vi "Waveform Channel Level.vi"(8 "error in (no error)":errorcluster, 11 "Node Ptr":T1 format="%.0x") -> (0 "error out":errorcluster)   [LabVIEW 2023, in "Embedded TDMS Logger System Explorer.lvlib"]
uses:
  Embedded TDMS Logger System Explorer.lvlib
  <vilib>/NI VeriStand/Custom Device API/Custom Device Item Ref.ctl
  Shared/Meta Data Item.ctl
  <vilib>/NI VeriStand/Custom Device API/Get Item Property (Dependent Node Pointer).vi
  <vilib>/NI VeriStand/Custom Device API/Set Item Property (Dependent Node Pointer).vi
  <vilib>/NI VeriStand/Custom Device API/Get Item Property (Variant).vi
  <vilib>/NI VeriStand/Custom Device API/Set Item Property (Variant).vi
  NationalInstruments.VeriStand.SystemStorage
  <vilib>/NI VeriStand/Custom Device API/Custom Device API.lvlib
  Shared/Embedded TDMS Logger Shared.lvlib
  <vilib>/NI VeriStand/Custom Device Tools/Custom Device Utility Library/Custom Device Utility Library.lvlib
panel:
  in  "Channel":string(combo)
  in  "Group Level Meta Data":string[][](table)
  in  "Specific Header":cluster{"Section Name":string}={"Section Name"="Specific Page Settings"}
  in  "General Header":cluster{"Section Name":string}={"Section Name"="General Page Settings"}
  in  "Description":string
  in  "Channel Name":string
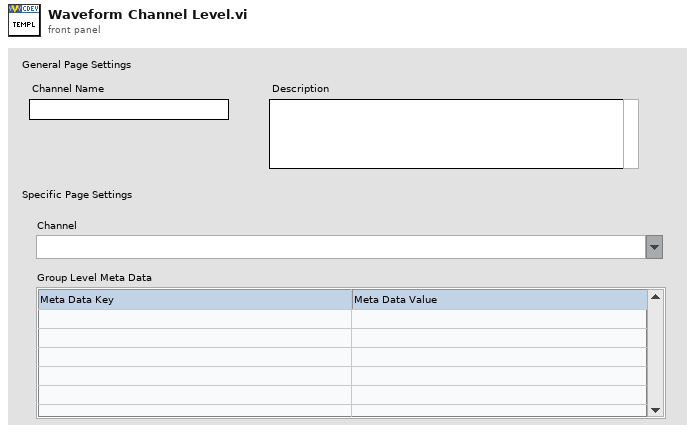
[diagram p1: front panel]
types:
  T1 = typedef "Custom Device API.lvlib/Custom Device Item Ref.ctl" = u64
  T2 = typedef "Embedded TDMS Logger Shared.lvlib/Meta Data Item.ctl" = cluster{"Key":string, "Value":string}
  T3 = typedef "Custom Device API.lvlib/Custom Device Pointer.ctl" = refnum<k24>
  T4 = typedef "Custom Device API.lvlib/Custom Device Item Info.ctl" = cluster{"Name":string, "Is Channel":bool, "GUID":string, "Is Waveform":bool}
  T5 = typedef "Custom Device API.lvlib/Custom Device Commands.ctl" = enum16{"Default", "Item renamed", "Shutdown", "Dynamic button pressed"}
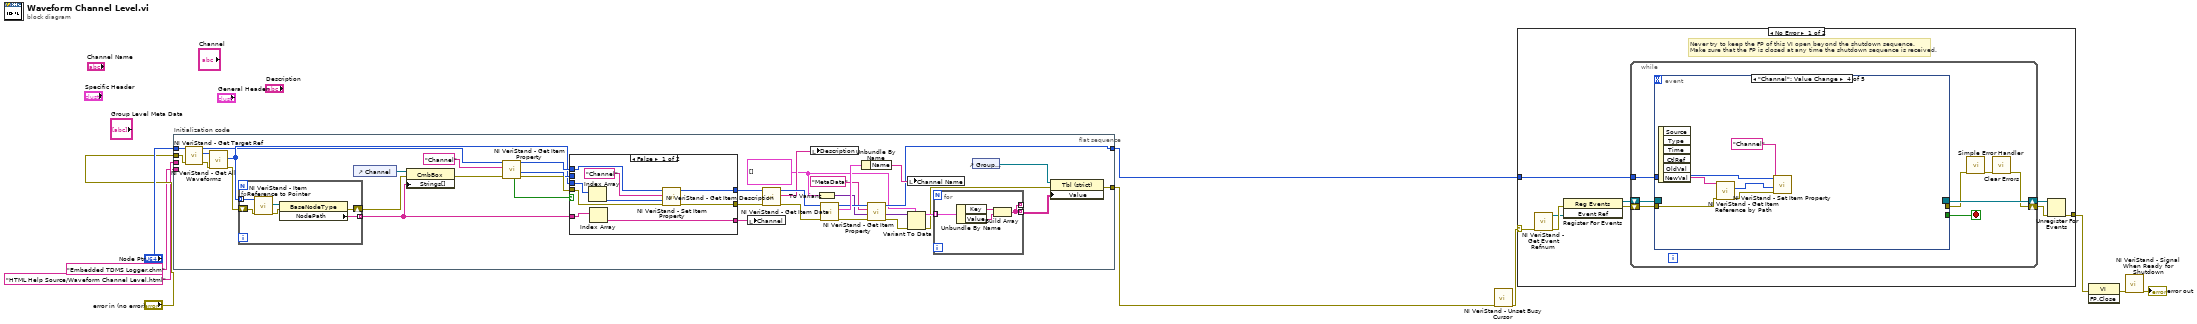
[diagram p0: block diagram]
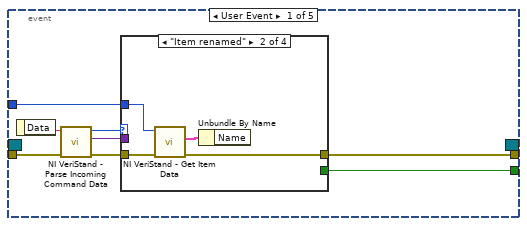
[diagram p2: hidden frame]
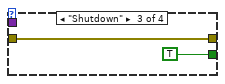
[diagram p4: hidden frame]
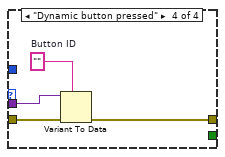
[diagram p5: hidden frame]
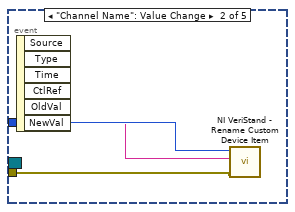
[diagram p6: hidden frame]
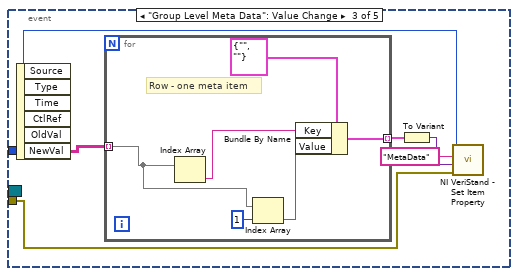
[diagram p7: hidden frame]
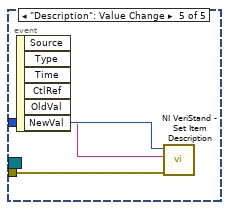
[diagram p8: hidden frame]
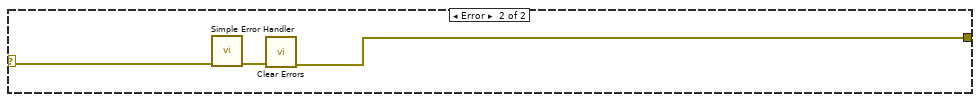
[diagram p9: hidden frame]
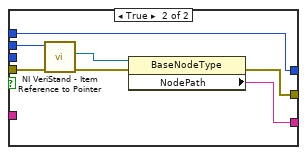
[diagram p10: hidden frame]
diagram:
  n1 = flat-sequence "Initialization code" {
    tunnel: "error in (no error)" -> [w39]
    tunnel: "Node Ptr" -> [w38]
    tunnel: [w24] -> w6
    tunnel: [w33] -> w3
    tunnel: "HTML Help Source/Waveform Channel Level.html" ("CD_CHM_Section") -> [_]
    tunnel: "Embedded TDMS Logger.chm" ("CD_CHM_FileName") -> [_]
    frame #0 {
      w29 = T2[] []
      n2 = call <vilib>:"NI VeriStand - Get Target Ref.vi"("error in"=w39, "Item Ref in"=w38) -> ("error out"=w40:errorcluster, "Target Ref"=w11:T1, "Item Ref out"=w12:T1)  [unwired: 6 in, 1 out]
      n3 = call <vilib>:"NI VeriStand - Get All Waveforms.vi"("error in"=w40, "Section Ref in"=w11) -> ("error out"=w41:errorcluster, "Waveform Refs"=w13:T1[])  [unwired: 6 in, 2 out]
      n4 = for {
        tunnel: w13 -> [w73] mode=indexing
        shift-right: [w68] -> w37
        shift-left: w41 -> [w72]
        tunnel: [w69] -> w18 mode=indexing
        n5 = call <vilib>:"NI VeriStand - Item Reference to Pointer.vi"("error in (no error)"=w72, "Item Ref in"=w73) -> ("error out"=w71:errorcluster, "Node Pointer"=w70:T3)  [unwired: 6 in, 2 out]
        n6 = property class="BaseNodeType"(reference=w70, error in=w71) -> (error out=w68:errorcluster, "NodePath"=w69:string)  [unwired: 1 out]
      }
      n7 = control-ref of="Channel"() -> (w42:refnum<vi>)
      n8 = property class="CmbBox"(reference=w42, error in=w37, "Strings[]"=w18) -> (error out=w14:errorcluster)  [unwired: 1 out]
      n9 = call-poly <vilib>:"NI VeriStand - Get Item Property.vi"("error in (no error)"=w14, "Property Name"="Channel", "Item Ref in"=w12) -> ("error out"=w22:errorcluster, "Dependent Node Ref"=w21:T1, "Item Ref out"=w20:T1, "Found"=w19:bool)  [unwired: 5 in]
      n10 = case shown="False" w19 {
        tunnel: w21 -> [_ w61]
        tunnel: w22 -> [w54 w60]
        tunnel: [w53 w59] -> w16
        tunnel: [w51 w58] -> w17
        tunnel: w20 -> [w55 w57]
        tunnel: w18 -> [w52 _]
        tunnel: [w50 w57] -> w15
        tunnel: w13 -> [w49 _]
        frame False {
          n11 = Index Array(array=w49) -> (element=w48:T1)  [unwired: 1 in]
          n12 = Index Array(array=w52) -> (element=w51:string)  [unwired: 1 in]
          n13 = call-poly <vilib>:"NI VeriStand - Set Item Property.vi"("error in (no error)"=w54, "Dependent Node Ref"=w48, "Property Name"="Channel", "Item Ref in"=w55) -> ("error out"=w53:errorcluster, "Item Ref out"=w50:T1)  [unwired: 5 in, 1 out]
        }
        frame True {
          n14 = call <vilib>:"NI VeriStand - Item Reference to Pointer.vi"("error in (no error)"=w60, "Item Ref in"=w61) -> ("error out"=w62:errorcluster, "Node Pointer"=w63:T3)  [unwired: 6 in, 2 out]
          n15 = property class="BaseNodeType"(reference=w63, error in=w62) -> (error out=w59:errorcluster, "NodePath"=w58:string)  [unwired: 1 out]
        }
      }
      n16 = local write "Channel"(w17) -> ()
      n17 = call <vilib>:"NI VeriStand - Get Item Description.vi"("error in (no error)"=w16, "Item Ref in"=w15) -> ("error out"=w46:errorcluster, "Description"=w43:string, "Item Ref out"=w47:T1)  [unwired: 7 out]
      n18 = local write "Description"(w43) -> ()
      n19 = To Variant(anything=w29) -> (Variant=w32:variant)
      n20 = call <vilib>:"NI VeriStand - Get Item Data.vi"("error in (no error)"=w46, "Item Ref in"=w47) -> ("error out"=w36:errorcluster, "Item Info"=w45:T4, "Item Ref out"=w35:T1)  [unwired: 7 out]
      n21 = Unbundle By Name(w45) -> ("Name"=w44:string)
      n22 = call-poly <vilib>:"NI VeriStand - Get Item Property.vi"("error in (no error)"=w36, "Default Value"=w32, "Property Name"="MetaData", "Item Ref in"=w35) -> ("error out"=w31:errorcluster, "Value"=w30:variant, "Item Ref out"=w33:T1)  [unwired: 4 in, 1 out]
      n23 = local write "Channel Name"(w44) -> ()
      n24 = Variant To Data(error in=w31, type=w29, Variant=w30) -> (data=w28:T2[], error out=w25:errorcluster)
      n25 = for {
        tunnel: w28 -> [w67] mode=indexing
        tunnel: [w64] -> _ mode=indexing
        tunnel: [w64] -> w26 mode=indexing
        n26 = Unbundle By Name(w67) -> ("Key"=w66:string, "Value"=w65:string)
        n27 = Build Array(w66, w65) -> (w64:string[])
      }
      n28 = control-ref of="Group Level Meta Data"() -> (w27:refnum<vi>)
      n29 = property class="Tbl (strict)"(reference=w27, error in=w25, "Value"=w26) -> (error out=w24:errorcluster)  [unwired: 1 out]
    }
  }
  n30 = call <vilib>:"NI VeriStand - Unset Busy Cursor.vi"("error in (no error)"=w6) -> ("error out"=w5:errorcluster)  [unwired: 10 out]
  n31 = case shown="No Error" w5 {
    selector: w5 -> [w74 w136]
    tunnel: [w79 w134] -> w10
    tunnel: w3 -> [w75 _]
    frame No Error {
      # "Never try to keep the FP of this VI open beyond the shutdown sequence.\nMake sure that the FP is closed at any time the shutdown sequence is received."
      n32 = call <vilib>:"NI VeriStand - Get Event Refnum.vi"("error in (no error)"=w74) -> ("error out"=w82:errorcluster, "Event Ref"=w78:refnum<user-event>)  [unwired: 9 out]
      n33 = register-events(error in=w82, w78) -> (reference out=w76:refnum<event-registration>, error out=w77:errorcluster)  [unwired: 1 in]
      n34 = while {
        tunnel: w75 -> [w86]
        shift-right: [w83] -> w80
        shift-left: w77 -> [w89]
        shift-right: [w90] -> w81
        shift-left: w76 -> [w88]
        stop <- w87 stop-if-true
        n35 = event shown="[3] \"Channel\": Value Change" {
          selector: w88 -> [_ _ _ _ _]
          dyn-events: [_ _ _ _ _] -> w90
          timeout: _ -> [_ _ _ _ _]
          tunnel: w89 -> [w98 w110 w113 w127 w132]
          tunnel: [w94 _ _ _ _] -> w87
          tunnel: [w93 _ _ _ _] -> w85
          tunnel: w86 -> [w92 w112 w114 w126 w133]
          event User Event {
            n36 = event-data() -> ("Data"=w97:string)  [unwired: 1 out]
            n37 = call <vilib>:"NI VeriStand - Parse Incoming Command Data.vi"("error in (no error)"=w98, "Incoming data"=w97) -> ("error out"=w96:errorcluster, "Outgoing data"=w91:variant, "Action"=w95:T5)  [unwired: 7 out]
            n38 = case shown="\"Item renamed\"" w95 {
              tunnel: w96 -> [w99 w103 w104 w109]
              tunnel: [_ _ TRUE _] -> w94
              tunnel: [w99 w100 w104 w106] -> w93
              tunnel: w92 -> [_ w102 _ _]
              tunnel: w91 -> [_ _ _ w108]
              frame "Default", Default {
              }
              frame "Item renamed" {
                n39 = call <vilib>:"NI VeriStand - Get Item Data.vi"("error in (no error)"=w103, "Item Ref in"=w102) -> ("error out"=w100:errorcluster, "Item Info"=w101:T4)  [unwired: 8 out]
                n40 = Unbundle By Name(w101) -> ()  [unwired: 1 out]
              }
              frame "Shutdown" {
              }
              frame "Dynamic button pressed" {
                w107 = ""  # Button ID
                n41 = Variant To Data(error in=w109, type=w107, Variant=w108) -> (error out=w106:errorcluster)  [unwired: 1 out]
              }
            }
          }
          event "Channel Name": Value Change {
            n42 = event-data() -> ("NewVal"=w111:string)  [unwired: 6 out]
            n43 = call <vilib>:"NI VeriStand - Rename Custom Device Item.vi"("error in (no error)"=w110, "New Name"=w111, "Item Ref in"=w112) -> ()  [unwired: 6 in, 3 out]
          }
          event "Group Level Meta Data": Value Change {
            n44 = event-data() -> ("NewVal"=w115:string[][])  [unwired: 6 out]
            n45 = for {
              tunnel: w115 -> [w123] mode=indexing
              tunnel: [w119] -> w118 mode=indexing
              # "Row - one meta item"
              n46 = Index Array(array=w123) -> (element=w120:string)  [unwired: 1 in]
              n47 = Index Array(array=w123, index=1) -> (element=w121:string)
              n48 = Bundle By Name(cluster=T2 {"Key"="", "Value"=""} ("Meta Data"), "Key"=w120, "Value"=w121) -> (w119:T2)
            }
            n49 = To Variant(anything=w118) -> (Variant=w117:variant)
            n50 = call-poly <vilib>:"NI VeriStand - Set Item Property.vi"("error in (no error)"=w113, "Value"=w117, "Property Name"="MetaData", "Item Ref in"=w114) -> ()  [unwired: 5 in, 3 out]
          }
          event "Channel": Value Change {
            n51 = event-data() -> ("NewVal"=w130:string)  [unwired: 6 out]
            n52 = call <vilib>:"NI VeriStand - Get Item Reference by Path.vi"("error in (no error)"=w127, "Item Path in"=w130) -> ("error out"=w128:errorcluster, "Item Ref"=w129:T1)  [unwired: 6 in, 2 out]
            n53 = call-poly <vilib>:"NI VeriStand - Set Item Property.vi"("error in (no error)"=w128, "Dependent Node Ref"=w129, "Property Name"="Channel", "Item Ref in"=w126) -> ()  [unwired: 5 in, 3 out]
          }
          event "Description": Value Change {
            n54 = event-data() -> ("NewVal"=w131:string)  [unwired: 6 out]
            n55 = call <vilib>:"NI VeriStand - Set Item Description.vi"("error in (no error)"=w132, "Description"=w131, "Item Ref in"=w133) -> ()  [unwired: 9 out]
          }
        }
        n56 = call <vilib>:"Simple Error Handler.vi"("error in (no error)"=w85) -> ("error out"=w84:errorcluster)  [unwired: 1 in, 7 out]
        n57 = call <vilib>:"Clear Errors.vi"("error in (no error)"=w84) -> ("error out"=w83:errorcluster)  [unwired: 1 in, 5 out]
      }
      n58 = Unregister For Events(event registration refnum=w81, error in=w80) -> (error out=w79:errorcluster)
    }
    frame Error {
      n59 = call <vilib>:"Simple Error Handler.vi"("error in (no error)"=w136) -> ("error out"=w135:errorcluster)  [unwired: 1 in, 7 out]
      n60 = call <vilib>:"Clear Errors.vi"("error in (no error)"=w135) -> ("error out"=w134:errorcluster)  [unwired: 1 in, 5 out]
    }
  }
  n61 = invoke class="VI" method="FP.Close"(error in=w10) -> (error out=w9:errorcluster)  [unwired: 2 in, 2 out]
  n62 = call <vilib>:"NI VeriStand - Signal When Ready for Shutdown.vi"("error in (no error)"=w9) -> ("error out"=→"error out":errorcluster)  [unwired: 10 out]
